vi "Error Query.vi"(8 "error in (no error)":errorcluster, 11 "VISA resource name":refnum<visa-resource-name>) -> (0 "error out":errorcluster, 1 "Error Message":string, 2 "Error Code":i32[](array[numeric]), 3 "VISA resource name out":refnum<visa-resource-name>)   [LabVIEW 2020, in "Active Technologies AWG3000.lvlib"]
doc: "Queries the instrument for any errors in the instrument's error queue. It will continue to read errors until all errors have been read from the instrument. Any errors will be returned in the <B>error out</B> control.\n\n<B>Note:</B>\n\nThis VI is called automatically by most driver VIs so it is not usually necessary to call this in an application."
uses:
  Active Technologies AWG3000.lvlib
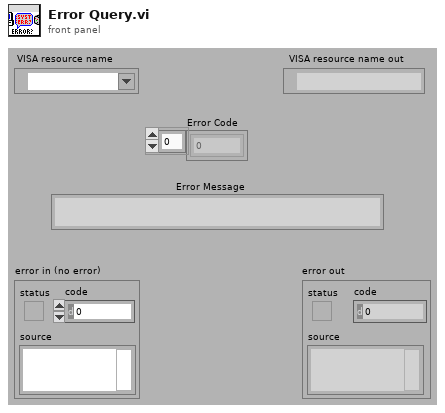
[diagram p1: front panel]
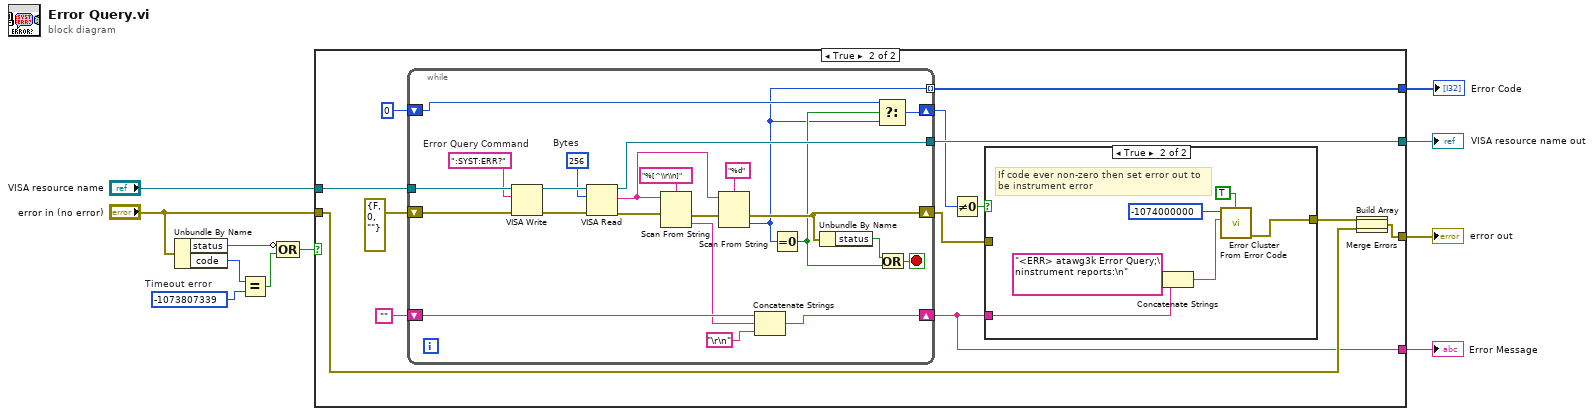
[diagram p0: block diagram]
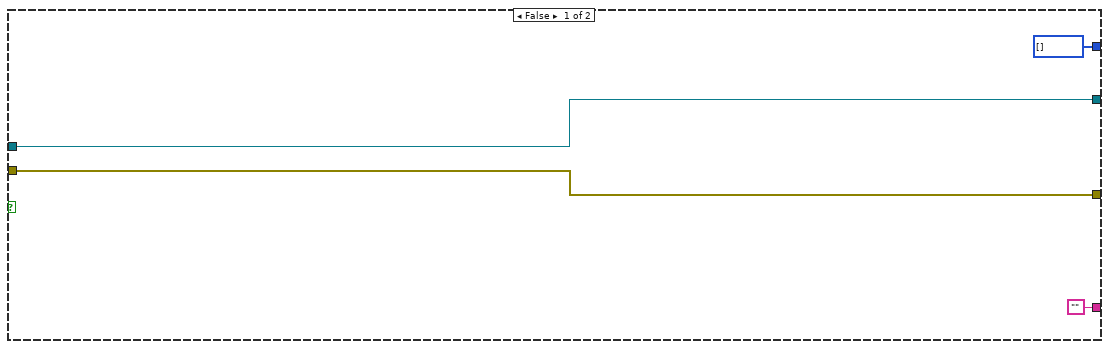
[diagram p2: hidden frame]
diagram:
  w6 = -1073807339  # Timeout error
  n1 = Unbundle By Name("error in (no error)") -> ("status"=w7:bool, "code"=w4:i32)
  n2 = Equal?(x=w4, y=w6) -> (x = y?=w5:bool)
  n3 = Compound Arithmetic op=OR(invert w7, w5) -> (w3:bool)
  n4 = case shown="True" w3 {
    tunnel: [w15 w29] -> w11
    tunnel: "VISA resource name" -> [w15 w28]
    tunnel: "error in (no error)" -> [w14 w22]
    tunnel: [w14 w26] -> w9
    tunnel: ["" w19] -> w2
    tunnel: [i32[] [] w18] -> w1
    frame False {
    }
    frame True {
      n5 = while {
        tunnel: [w59] -> w29
        tunnel: w28 -> [w58]
        shift-right: [w46] -> w19
        shift-left: "" -> [w49]
        shift-right: [w44] -> w20
        shift-left: 0 -> [w45]
        shift-right: [w42] -> w17
        shift-left: errorcluster {"status"=FALSE, "code"=0, "source"=""} ("error in (no error)") -> [w43]
        tunnel: [w37] -> w18 mode=indexing
        stop <- w52 stop-if-true
        w56 = u32 256  # Bytes
        w54 = ":SYST:ERR?"  # Error Query Command
        n6 = VISA Write(VISA resource name=w58, write buffer=w54, error in (no error)=w43) -> (VISA resource name out=w57:refnum<visa-resource-name>, error out=w55:errorcluster)  [unwired: 1 out]
        n7 = VISA Read(VISA resource name=w57, byte count=w56, error in (no error)=w55) -> (VISA resource name out=w59:refnum<visa-resource-name>, read buffer=w50:string, error out=w41:errorcluster)  [unwired: 1 out]
        n8 = Scan From String(format string="%[^\\r\\n]", input string=w50, error in=w41) -> (error out=w40:errorcluster, output 1=w47:string)  [unwired: 2 in, 2 out]
        n9 = Scan From String(format string="%d", input string=w50, error in=w40) -> (error out=w42:errorcluster, output 1=w37:i32)  [unwired: 2 in, 2 out]
        n10 = Concatenate Strings(w49, w47, "\r\n") -> (w46:string)
        n11 = Equal To 0?(x=w37) -> (x = 0?=w38:bool)
        n12 = Unbundle By Name(w42) -> ("status"=w39:bool)
        n13 = Select(t=w45, s=w38, f=w37) -> (s? t:f=w44:i32)
        n14 = Or(x=w39, y=w38) -> (x .or. y?=w52:bool)
      }
      n15 = Not Equal To 0?(x=w20) -> (x != 0?=w24:bool)
      n16 = case shown="True" w24 {
        tunnel: w19 -> [_ w35]
        tunnel: [w30 w34] -> w23
        tunnel: w17 -> [w30 _]
        frame False {
        }
        frame True {
          # "If code ever non-zero then set error out to\nbe instrument error"
          n17 = Concatenate Strings("<ERR> atawg3k Error Query;\ninstrument reports:\n" ("Source"), w35) -> (w31:string)
          n18 = call <vilib>:"Error Cluster From Error Code.vi"("show call chain? (False)"=TRUE ("Status"), "error message (\"\")"=w31, "error code (0)"=-1074000000 ("Code")) -> ("error out"=w34:errorcluster)  [unwired: 6 in]
        }
      }
      n19 = Build Array(w23, w22) -> (w16:errorcluster[])
      n20 = Merge Errors(w16) -> (w26:errorcluster)
    }
  }
  "VISA resource name out" <- w11
  "error out" <- w9
  "Error Message" <- w2
  "Error Code" <- w1
